vi "Test UI.vi"() -> ()   [LabVIEW 2012]
panel:
  out "timestamp":timestamp
  in  "Boolean":bool
  out "Waveform Graph":sgl[](graph)
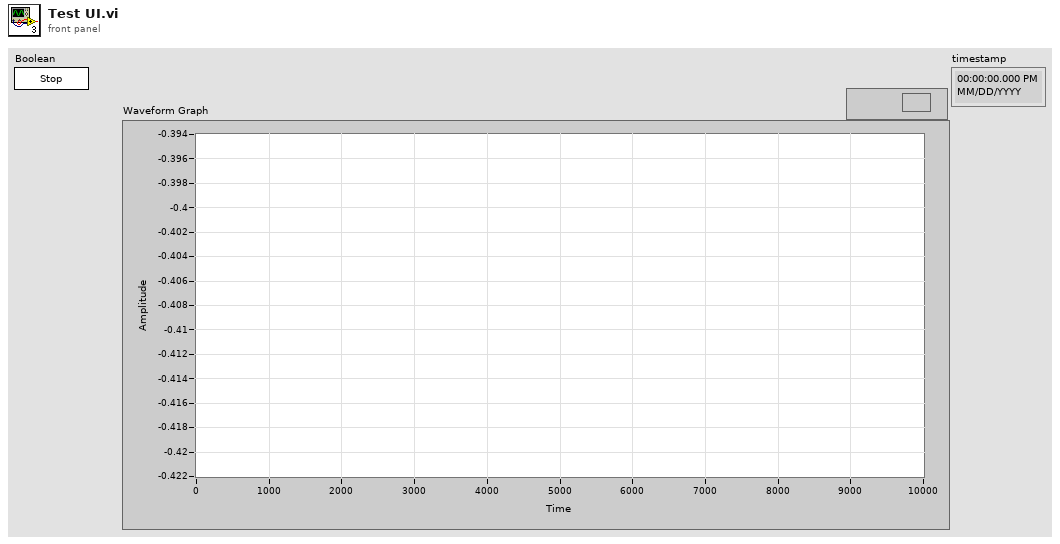
[diagram p1: front panel]
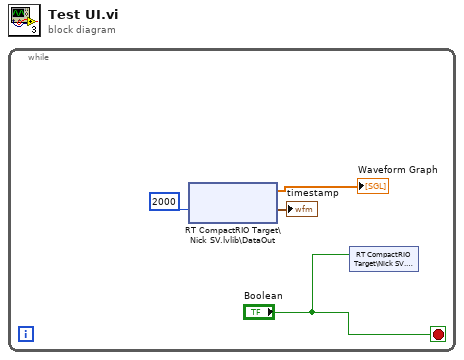
[diagram p0: block diagram]
diagram:
  n1 = while {
    stop <- "Boolean" stop-if-true
    n2 = shared-variable "RT CompactRIO Target\\Nick SV.lvlib\\DataOut"(2000 ("ms timeout (0)")) -> (→"Waveform Graph":sgl[], →"timestamp":timestamp)  [unwired: 1 in, 2 out]
    n3 = shared-variable "RT CompactRIO Target\\Nick SV.lvlib\\Stop"("Boolean") -> ()  [unwired: 1 in, 1 out]
  }
